vi "CC convert angle to SS and MM.vi"(10 "Angle":dbl) -> (1 "Minutes":dbl, 2 "Seconds":dbl)   [LabVIEW 2024]
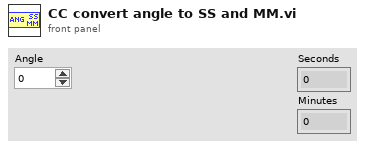
[diagram p1: front panel]
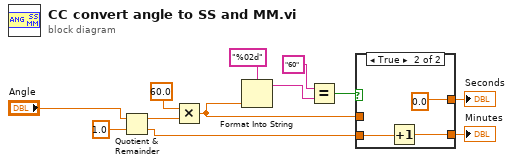
[diagram p0: block diagram]
diagram:
  n1 = Quotient & Remainder(x="Angle", y=1.0) -> (x-y*floor(x/y)=w6:dbl, floor(x/y)=w4:dbl)
  n2 = Multiply(x=60.0 ("y"), y=w6) -> (x*y=w3:dbl)
  n3 = Format Into String(format string="%02d", w3) -> (resulting string=w9:string)  [unwired: 2 in, 1 out]
  n4 = Equal?(x="60", y=w9) -> (x = y?=w11:bool)
  n5 = case shown="True" w11 {
    tunnel: w4 -> [w13 w17]
    tunnel: [w14 0.0] -> w2
    tunnel: [w13 w15] -> w1
    tunnel: w3 -> [w14 _]
    frame False {
    }
    frame True {
      n6 = Increment(x=w17) -> (x+1=w15:dbl)
    }
  }
  "Seconds" <- w2
  "Minutes" <- w1
